vi "RUC_measurment(F-x-V-I).vi"() -> ()   [LabVIEW 2018]
panel:
  out "Current [V]":dynamicdata(graph)
  out "Voltage [V]":dynamicdata(graph)
  in  "Filename":path=path "C:/Users/Bizjan/Desktop/Structural dynamics of 3D printed thermoactive metamaterials/Measurements/RUC_measunments/test.lvm"
  out "F(x) [N/mm]":cluster{"Y":dbl[], "Y":dbl[]}[](graph)
  out "Pomik x [mm]":dynamicdata(graph)
  out "Sila F [N]":dynamicdata(graph)
  in  "Enable":bool=TRUE
  in  "stop (F)":bool
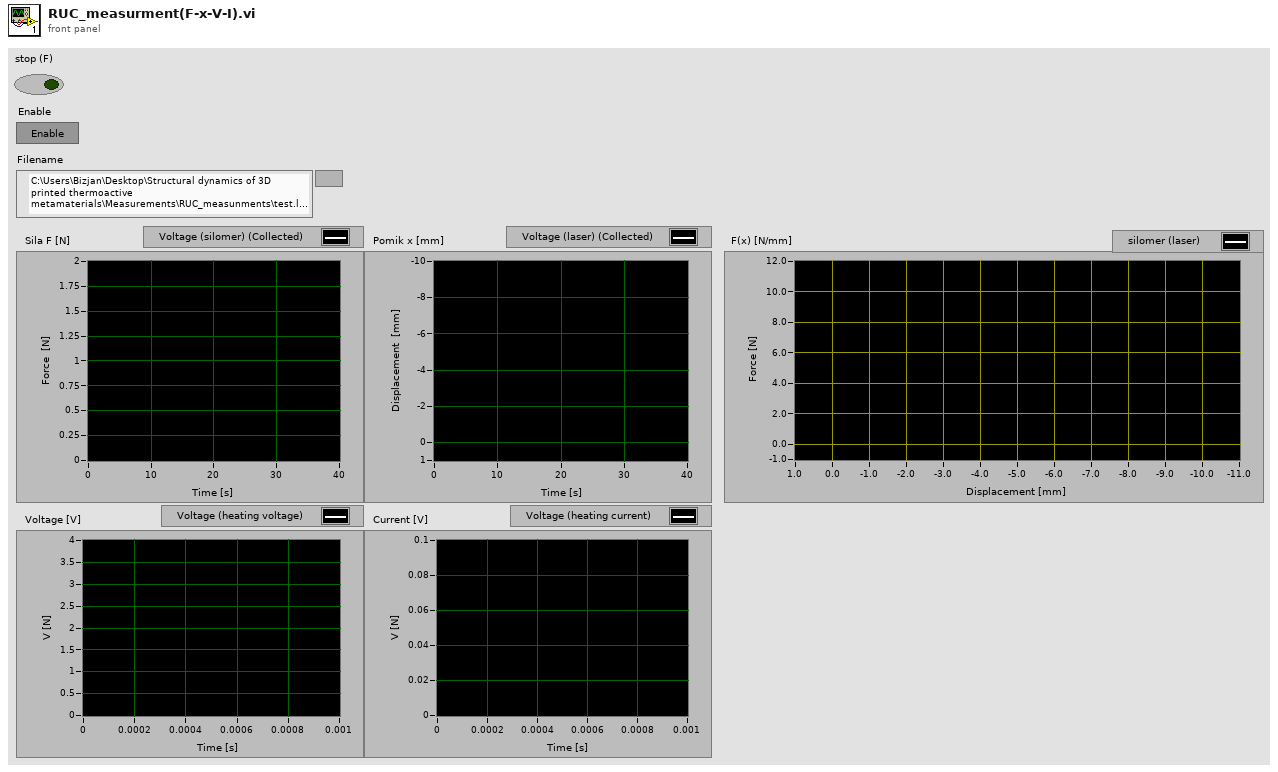
[diagram p1: front panel]
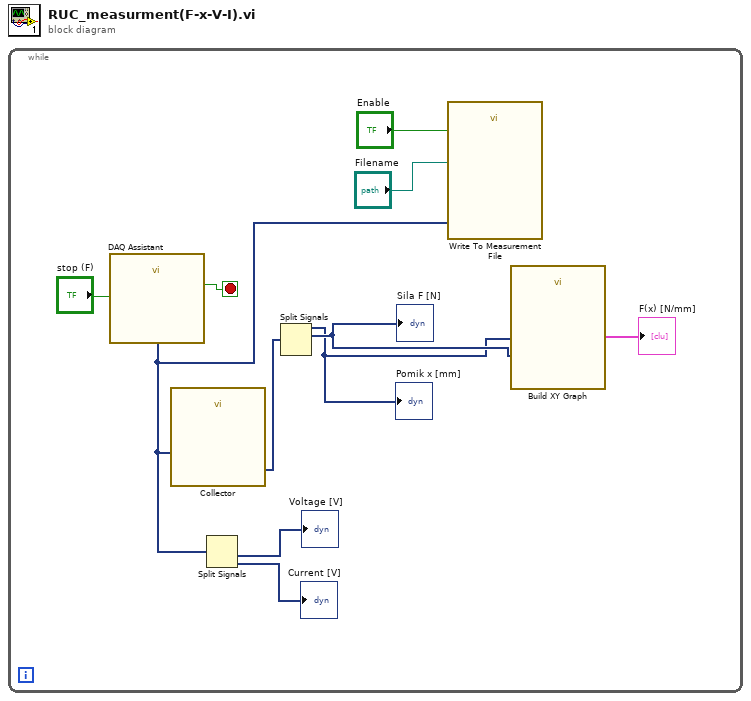
[diagram p0: block diagram]
diagram:
  n1 = while {
    stop <- w9 stop-if-true
    n2 = call "DAQ Assistant"("stop (F)"="stop (F)") -> ("data"=w1:dynamicdata, "stopped"=w9:bool)  [unwired: 15 in, 2 out]
    n3 = call "Collector"("Signals"=w1) -> ("Collected Signals"=w6:dynamicdata)  [unwired: 9 in, 1 out]
    n4 = Split Signals(w1) -> (→"Voltage [V]":dynamicdata, →"Current [V]":dynamicdata)  [unwired: 4 in, 2 out]
    n5 = Split Signals(w6) -> (w7:dynamicdata, w8:dynamicdata)  [unwired: 4 in, 2 out]
    "Sila F [N]" <- w8
    "Pomik x [mm]" <- w7
    n6 = call "Write To Measurement File"("Signals"=w1, "Enable"="Enable", "Filename"="Filename") -> ()  [unwired: 14 in, 3 out]
    n7 = call "Build XY Graph"("Y Input"=w8, "X Input"=w7) -> ("XY Graph"=→"F(x) [N/mm]":cluster{"X":dbl[], "Y":dbl[]}[])  [unwired: 8 in, 1 out]
  }
